vi "Control_BIG.vi"() -> ()   [LabVIEW 2017]
uses:
  <vilib>/myRIO/Common/Instrument Driver Framework/myRIO v1.0/UART/vis/myRIO v1.0 Close UART.vi
  <vilib>/FPGAPlugInAG/myRIO-1900/niLvFpga_Open_myRIO-1900.vi
  <vilib>/rvi/interface/common/dynamic/niFpgaDynamicAddResources.vi
  <vilib>/myRIO/Common/Instrument Driver Framework/Utilities/vis/FPGA Ref Manager.vi
  <vilib>/Utility/error.llb/Error Cluster From Error Code.vi
  <vilib>/myRIO/Common/Instrument Driver Framework/Utilities/vis/Ref Counter.vi
  <vilib>/FPGAPlugInAG/Dynamic/niLvFpga_Close_Dynamic.vi
  <vilib>/myRIO/Common/Instrument Driver Framework/myRIO v1.0/myRIO v1.0 Reset FPGA.vi
  <vilib>/myRIO/Common/Instrument Driver Framework/myRIO v1.0/IRQ/vis/myRIO v1.0 IRQ Info FGV.vi
  <vilib>/myRIO/Common/Instrument Driver Framework/myRIO v1.0/IRQ/vis/myRIO v1.0 Timer IRQ Info FGV.vi
  <vilib>/myRIO/Common/Instrument Driver Framework/myRIO v1.0/IRQ/vis/myRIO v1.0 ISR Agent.vi
  <vilib>/rvi/interface/nirviOpenFPGA/nirviOpenFPGA.xnode
  FPGA Bitfiles/Motor-Controller_FPGATarget_FPGAMainDefault_mthDGtjqrtg.lvbitx
  <vilib>/rvi/interface/nirviCloseFPGA/nirviCloseFPGA.xnode
  <vilib>/myRIO/Instrument Drivers/Utilities/Utilities.lvlib
panel:
  in  "Type":enum16{"Iterations", "Counts", "Time"}(ring)
  in  "Motor":T1(ring)=enum."A/Motor2"
  in  "Encoder":T2(ring)
  in  "Position":dbl(slide)=1.5 scale=0.8..2.2 scale format="%#_3g"
  in  "STOP":bool
  in  "Iteraciones":dbl
  out "Waveform Chart":dbl[][](graph)
  in  "Speed (Lower than 1200 counts/s)":dbl
  out "error out":errorcluster
  # "Programa que funciona para probar los bloques de motores.\nInteraciones: Punto final donde se quiere hacer llegar el motor.\nSpeed: Velocidad a la que se quiere correr el motor.\nChannel Name: Canal del PWM donde se controla el motor.\nError: Indicador de error al finalizar el programa.\nSTOP: Botón de parada del programa, siempre usar este, NUNCA \nDETENER EL PROGARMA CON ABORT EXCECUTION."
  # "Nota: El motor grande nunca llevarlo a más de 600 c/sec"
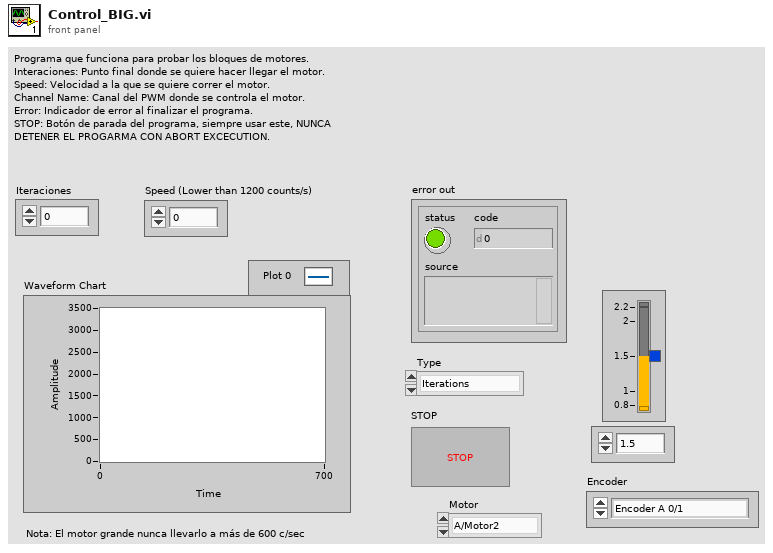
[diagram p1: front panel]
types:
  T1 = enum16{"B/Motor2", "B/Motor1", "A/Motor2", "A/Motor1"}
  T2 = enum16{"Encoder A 0/1", "Encoder A 11/12", "Encoder A 4/13", "Encoder B 0/1", "Encoder B 11/12", "Encoder B 4/13", "Encoder C 4/6", "Encoder C 0/2"}
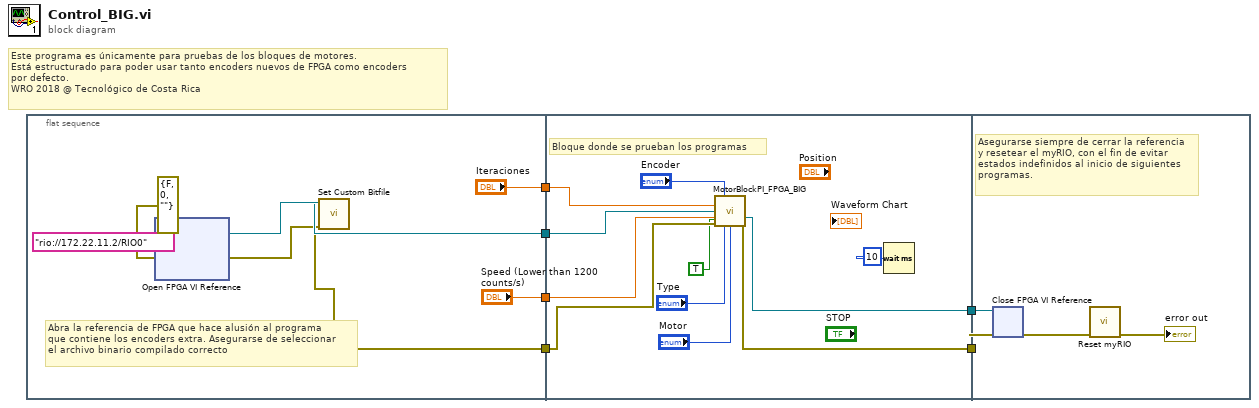
[diagram p0: block diagram]
diagram:
  # "Este programa es únicamente para pruebas de los bloques de motores.\nEstá estructurado para poder usar tanto encoders nuevos de FPGA como encoders \npor defecto.\nWRO 2018 @ Tecnológico de Costa Rica"
  n1 = flat-sequence {
    tunnel: [w7] -> w6
    tunnel: ["Iteraciones"] -> w5
    tunnel: ["Speed (Lower than 1200 counts/s)"] -> w4
    tunnel: [w9] -> w2
    tunnel: w6 -> [w20]
    tunnel: w5 -> [w23]
    tunnel: w4 -> [w21]
    tunnel: [w16] -> w3
    tunnel: w2 -> [w22]
    tunnel: [w15] -> w1
    tunnel: w3 -> [w27]
    tunnel: w1 -> [w28]
    frame #0 {
      # "Abra la referencia de FPGA que hace alusión al programa\nque contiene los encoders extra. Asegurarse de seleccionar\nel archivo binario compilado correcto"
      n2 = xnode "Open FPGA VI Reference"("error in"=errorcluster {"status"=FALSE, "code"=0, "source"=""}, "resource name"=tag "rio://172.22.11.2/RIO0") -> ("FPGA VI Reference Out"=w10:refnum<k20>, "error out"=w8:errorcluster)
      n3 = call <vilib>:"Set Custom Bitfile.vi"("error in (no error)"=w8, "Custom FPGA Reference In"=w10) -> ("error out"=w7:errorcluster, "Custom FPGA Reference Out"=w9:refnum<k20>)  [unwired: 8 in]
    }
    frame #1 {
      # "Bloque donde se prueban los programas"
      n4 = call "MotorBlockPI_FPGA_BIG.vi"("Encoder"="Encoder", "Value"=w23, "Custom FPGA Reference In"=w22, "Speed"=w21, "error in (no error)"=w20, "Type"="Type", "Motor"="Motor", "Sentido"=TRUE ("(Antihorario) Sentido (Horario)")) -> ("FPGA VI Reference Out"=w15:refnum<k20>, "error out"=w16:errorcluster)  [unwired: 5 in, 1 out]
      n5 = Wait (ms)(milliseconds to wait=u32 10) -> ()  [unwired: 1 out]
    }
    frame #2 {
      # "Asegurarse siempre de cerrar la referencia\ny resetear el myRIO, con el fin de evitar \nestados indefinidos al inicio de siguientes\nprogramas."
      n6 = xnode "Close FPGA VI Reference"("FPGA VI Reference In"=w28, "error in"=w27) -> ("error out"=w26:errorcluster)
      n7 = call <vilib>:"Reset myRIO.vi"("error in (no error)"=w26) -> ("error out"=→"error out":errorcluster)  [unwired: 10 in]
    }
  }
